vi "Make K-Points File, Manual.vi"(8 "K-point Mesh":T1(array[cluster]), 9 "# Points between":i32, 10 "Symmetry":enum32{"High-Symmetry", "L-G-X", "Manual Mesh"}(radio), 11 "Manual Type":enum32{"Reciprocal", "Cartesian"}(radio)) -> (3 "K-Points File":string)   [LabVIEW 2010]
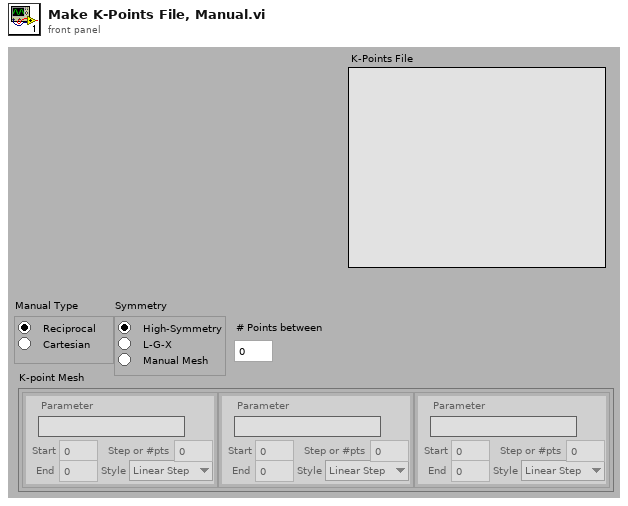
[diagram p1: front panel]
types:
  T1 = cluster{"Start":dbl, "End":dbl, "Step or #pts":dbl, "Style":enum16{"Linear Step", "Linear Pts", "Log Pts"}, "Parameter":string}[]
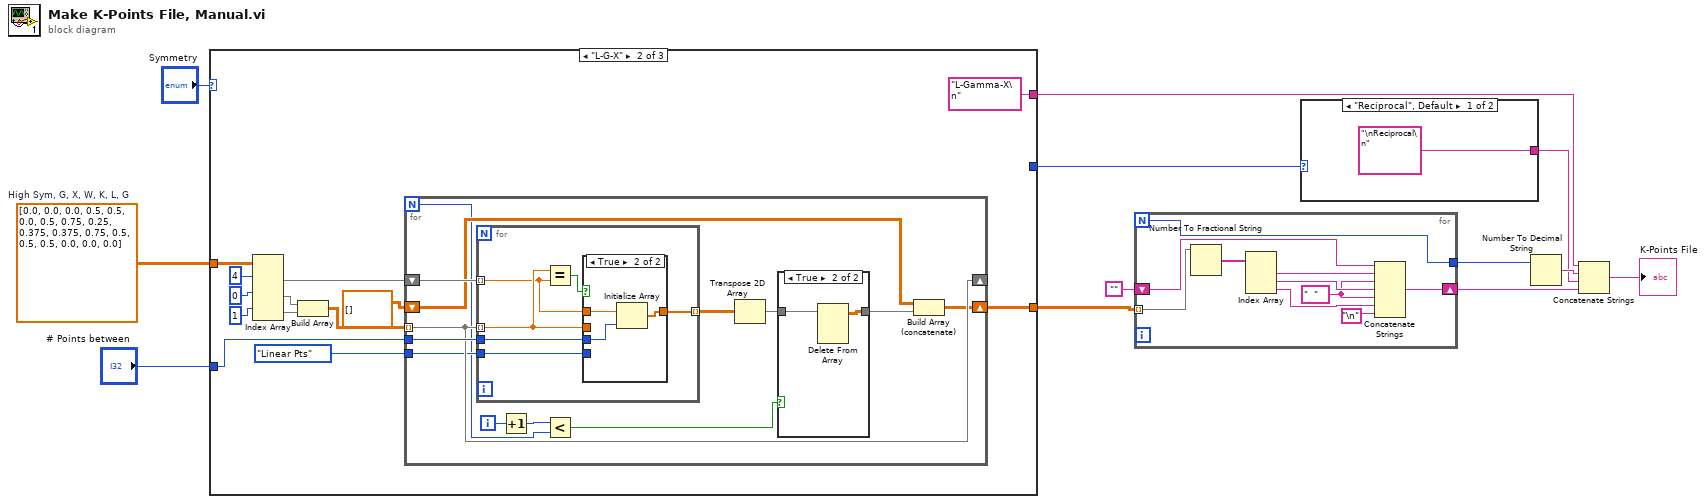
[diagram p0: block diagram]
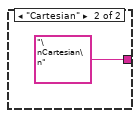
[diagram p2: hidden frame]
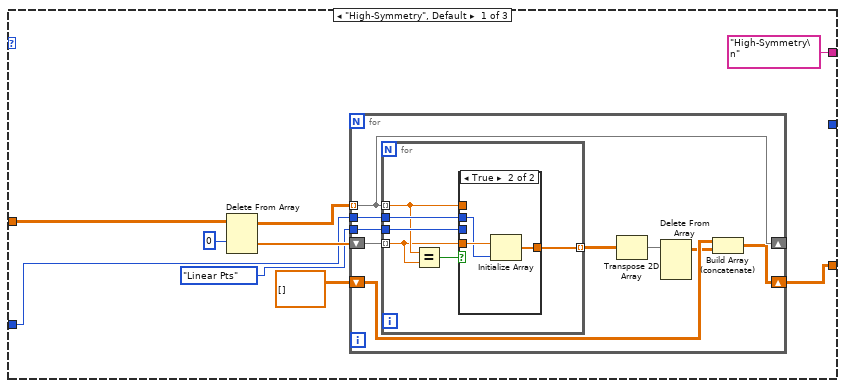
[diagram p3: hidden frame]
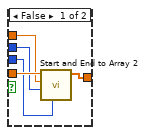
[diagram p4: hidden frame]
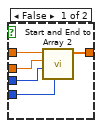
[diagram p6: hidden frame]
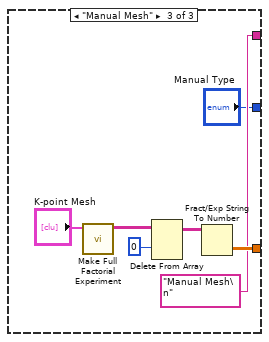
[diagram p7: hidden frame]
diagram:
  w10 = dbl[][] [[0.0, 0.0, 0.0], [0.5, 0.5, 0.0], [0.5, 0.75, 0.25], [0.375, 0.375, 0.75], [0.5, 0.5, 0.5], [0.0, 0.0, 0.0]]  # High Sym, G, X, W, K, L, G
  n1 = case shown="\"L-G-X\"" "Symmetry" {
    tunnel: w10 -> [w20 w47 _]
    tunnel: [w14 w54 w90] -> w8
    tunnel: "# Points between" -> [w16 w56 _]
    tunnel: ["High-Symmetry\n" "L-Gamma-X\n" "Manual Mesh\n"] -> w6
    tunnel: [_ _ "Manual Type"] -> w3
    frame "High-Symmetry", Default {
      n2 = Delete From Array(array=w20, index (row)=0) -> (deleted portion=w18:dbl[], array with subset deleted=w17:dbl[][])  [unwired: 2 in]
      n3 = for {
        shift-right: [w28] -> _
        shift-left: w18 -> [w30]
        shift-right: [w26] -> w14
        shift-left: dbl[][] [] -> [w25]
        tunnel: w17 -> [w28] mode=indexing
        tunnel: w16 -> [w29]
        tunnel: enum16{"Linear Step", "Linear Pts", "Log Pts"}."Linear Pts" ("Sweep Style") -> [w24]
        n4 = for {
          tunnel: w30 -> [w32] mode=indexing
          tunnel: w28 -> [w33] mode=indexing
          tunnel: w29 -> [w36]
          tunnel: [w35] -> w27 mode=indexing
          tunnel: w24 -> [w34]
          n5 = Equal?(x=w33, y=w32) -> (x = y?=w31:bool)
          n6 = case shown="True" w31 {
            tunnel: w32 -> [w41 w44]
            tunnel: w33 -> [w40 _]
            tunnel: w36 -> [w39 w43]
            tunnel: [w38 w42] -> w35
            tunnel: w34 -> [w37 _]
            frame False {
              n7 = call "Start and End to Array 2.vi"("Sweep Style"=w37, "Step or # Pts"=w39, "End"=w40, "Start"=w41) -> ("Array"=w38:dbl[])  [unwired: 7 in]
            }
            frame True {
              n8 = Initialize Array(w44, w43) -> (w42:dbl[])
            }
          }
        }
        n9 = Transpose 2D Array(2D array=w27) -> (transposed array=w23:dbl[][])
        n10 = Delete From Array(array=w23) -> (array with subset deleted=w22:dbl[][])  [unwired: 3 in, 1 out]
        n11 = Build Array (concatenate)(w25, w22) -> (w26:dbl[][])
      }
    }
    frame "L-G-X" {
      n12 = Index Array(array=w47, index (row) #1=4 ("index (row)"), index (row) #2=0 ("index (row)"), index (row) #3=1 ("index (row)")) -> (element #1=w46:dbl[], element #2=w49:dbl[], element #3=w48:dbl[])  [unwired: 3 in]
      n13 = Build Array(w49, w48) -> (w45:dbl[][])
      n14 = for {
        N -> [w59]
        shift-right: [w68] -> _
        shift-left: w46 -> [w70]
        shift-right: [w66] -> w54
        shift-left: dbl[][] [] -> [w65]
        tunnel: w45 -> [w68] mode=indexing
        tunnel: w56 -> [w69]
        tunnel: enum16{"Linear Step", "Linear Pts", "Log Pts"}."Linear Pts" ("Sweep Style") -> [w64]
        i -> [w61]
        n15 = for {
          tunnel: w70 -> [w75] mode=indexing
          tunnel: w68 -> [w76] mode=indexing
          tunnel: w69 -> [w79]
          tunnel: [w78] -> w67 mode=indexing
          tunnel: w64 -> [w77]
          n16 = Equal?(x=w76, y=w75) -> (x = y?=w74:bool)
          n17 = case shown="True" w74 {
            tunnel: w75 -> [w84 w87]
            tunnel: w76 -> [w83 _]
            tunnel: w79 -> [w82 w86]
            tunnel: [w81 w85] -> w78
            tunnel: w77 -> [w80 _]
            frame False {
              n18 = call "Start and End to Array 2.vi"("Sweep Style"=w80, "Step or # Pts"=w82, "End"=w83, "Start"=w84) -> ("Array"=w81:dbl[])  [unwired: 7 in]
            }
            frame True {
              n19 = Initialize Array(w87, w86) -> (w85:dbl[])
            }
          }
        }
        n20 = Increment(x=w61) -> (x+1=w60:i32)
        n21 = Less?(x=w60, y=w59) -> (x < y?=w58:bool)
        n22 = Transpose 2D Array(2D array=w67) -> (transposed array=w63:dbl[][])
        n23 = case shown="True" w58 {
          tunnel: w63 -> [w71 w73]
          tunnel: [w71 w72] -> w62
          frame False {
          }
          frame True {
            n24 = Delete From Array(array=w73) -> (array with subset deleted=w72:dbl[][])  [unwired: 3 in, 1 out]
          }
        }
        n25 = Build Array (concatenate)(w65, w62) -> (w66:dbl[][])
      }
    }
    frame "Manual Mesh" {
      n26 = call "Make Full Factorial Experiment.vi"("Array of Array Settings"="K-point Mesh") -> ("Full Factorial Design"=w93:string[][])  [unwired: 10 in]
      n27 = Delete From Array(array=w93, index (row)=0) -> (array with subset deleted=w91:string[][])  [unwired: 2 in, 1 out]
      n28 = Fract/Exp String To Number(string=w91) -> (number=w90:dbl[][])  [unwired: 3 in, 1 out]
    }
  }
  n29 = for {
    N -> [w95]
    tunnel: w8 -> [w104] mode=indexing
    shift-right: [w97] -> w1
    shift-left: "" -> [w96]
    tunnel: [w95] -> w5
    w100 = "  "
    n30 = Number To Fractional String(number=w104) -> (F-format string=w103:string[])  [unwired: 3 in]
    n31 = Index Array(array=w103) -> (element #1=w102:string, element #2=w101:string, element #3=w99:string)  [unwired: 3 in]
    n32 = Concatenate Strings(w96, w102, w100, w101, w100, w99, "\n") -> (w97:string)
  }
  n33 = case shown="\"Reciprocal\", Default" w3 {
    tunnel: ["\nReciprocal\n" "\nCartesian\n"] -> w2
    frame "Reciprocal", Default {
    }
    frame "Cartesian" {
    }
  }
  n34 = Number To Decimal String(number=w5) -> (decimal integer string=w4:string)  [unwired: 1 in]
  n35 = Concatenate Strings(w6, w4, w2, w1) -> (→"K-Points File":string)
